vi "ADO Connection Set Properties.vi"(8 "error in (no error)":errorcluster caption="错误输入（无错误）", 10 "connection properties":T1, 11 "Database Connection 输入":refnum<class "Database Connection.lvclass"> caption="DNL_LabVIEW Object in") -> (0 "error out":errorcluster caption="错误输出", 3 "Database Connection 输出":refnum<class "Database Connection.lvclass"> caption="DNL_LabVIEW Object out")   [LabVIEW 2011, in "Database Connection.lvclass"]
uses:
  Database Connection.lvclass
  Database Connection.lvclass/Database Connection.ctl
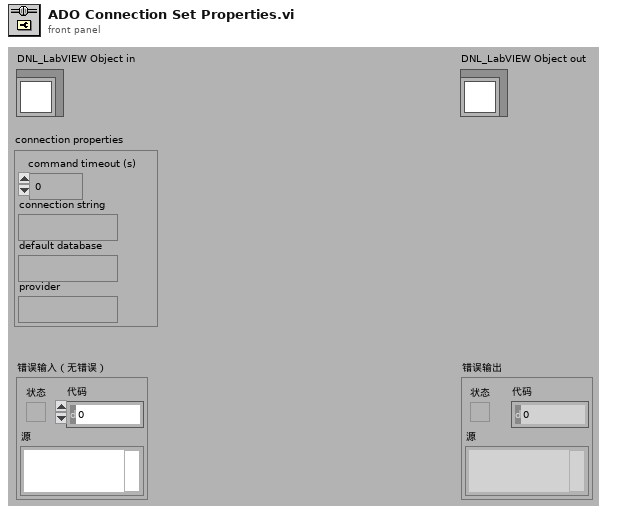
[diagram p1: front panel]
types:
  T1 = cluster{"command timeout (s)":i32, "connection string":string, "default database":string, "provider":string}
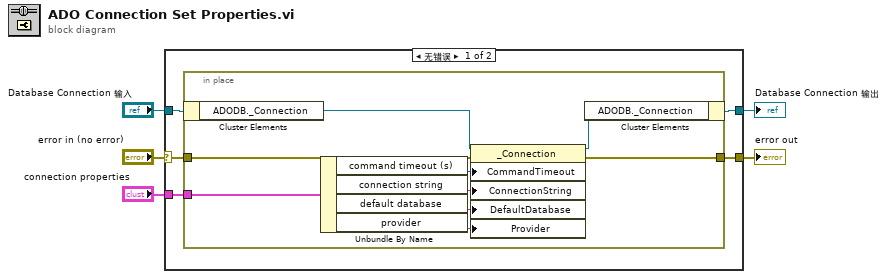
[diagram p0: block diagram]
diagram:
  n1 = case shown="无错误" "error in (no error)" {
    selector: "error in (no error)" -> [w9 w21]
    tunnel: [w8 w21] -> w4
    tunnel: [w6 w20] -> w2
    tunnel: "Database Connection 输入" -> [w10 w20]
    tunnel: "connection properties" -> [w7 _]
    frame No Error {
      n2 = in-place {
        in-place-border: w9 -> [w17]
        in-place-border: [w16] -> w8
        in-place-border: w7 -> [w11]
        n3 = in-place-cluster #1(w10) -> ("ADODB._Connection"=w19:refnum<k7>)
        n4 = Unbundle By Name(w11) -> ("command timeout (s)"=w15:i32, "connection string"=w14:string, "default database"=w13:string, "provider"=w12:string)
        n5 = property class="_Connection"(reference=w19, error in=w17, "CommandTimeout"=w15, "ConnectionString"=w14, "DefaultDatabase"=w13, "Provider"=w12) -> (reference out=w18:refnum<k7>, error out=w16:errorcluster)
        n6 = in-place-cluster #1("ADODB._Connection"=w18) -> (w6:refnum<class "Database Connection.lvclass">)
      }
    }
    frame Error {
    }
  }
  "error out" <- w4
  "Database Connection 输出" <- w2
